vi "Change Behavior IE window.vi"(7 "Front Panel Window:Behavior":T1(ring), 8 "error in (no error)":errorcluster, 11 "IE VI Ref":refnum<vi>) -> (0 "error out":errorcluster)   [LabVIEW 2021]
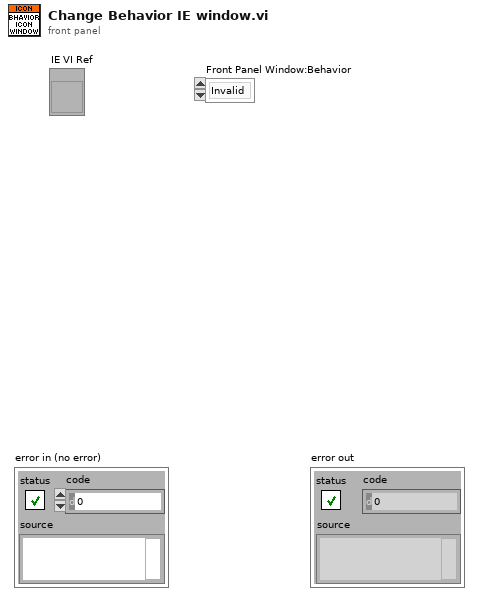
[diagram p1: front panel]
types:
  T1 = enum32{"Invalid", "Default", "Floating", "Floating/Auto-Hide", "Modal"}
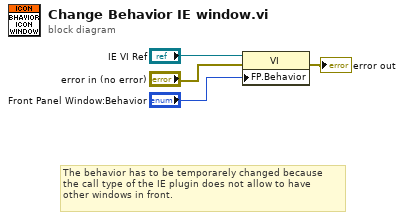
[diagram p0: block diagram]
diagram:
  # "The behavior has to be temporarely changed because\nthe call type of the IE plugin does not allow to have\nother windows in front."
  n1 = property class="VI"(reference="IE VI Ref", error in="error in (no error)", "FP.Behavior"="Front Panel Window:Behavior") -> (error out=→"error out":errorcluster)  [unwired: 1 out]
